vi "SetADGainGUI.vi"() -> ()   [LabVIEW 8.6]
uses:
  Program Files/National Instruments/LabVIEW 2010/resource/objmgr/daqmx.rc
panel:
  in  "select AI range":u16(ring) items=["-0.2 : 0.2 V", "-0.5 : 0.5 V", "-1.0 : 1.0 V", "-2.0 : 2.0 V", "-5.0 : 5.0 V", "-10.0 : 10.0 V", "-20.0 : 20.0 V", "-42.0 : 42.0 V"]
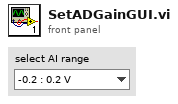
[diagram p1: front panel]
types:
  T1 = enum16{"None/#Datasets", "Clear", "TagValueOf#", "AddValues", "ReadValue", "ChangeValue", "Get all"}
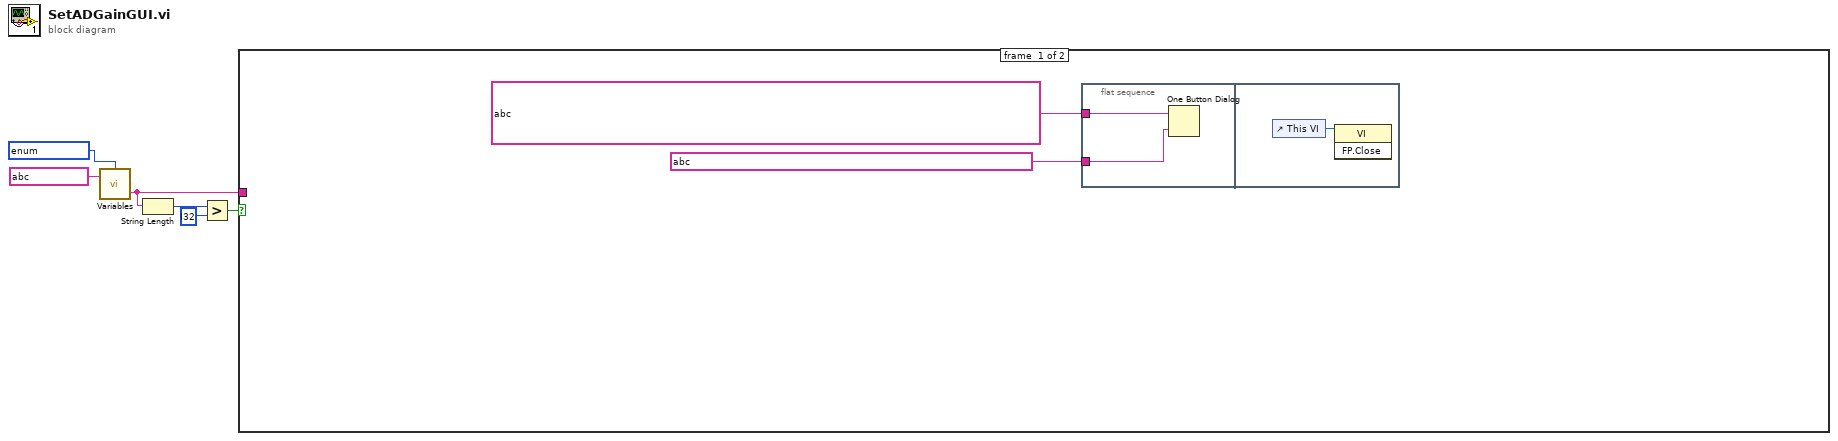
[diagram p0: block diagram]
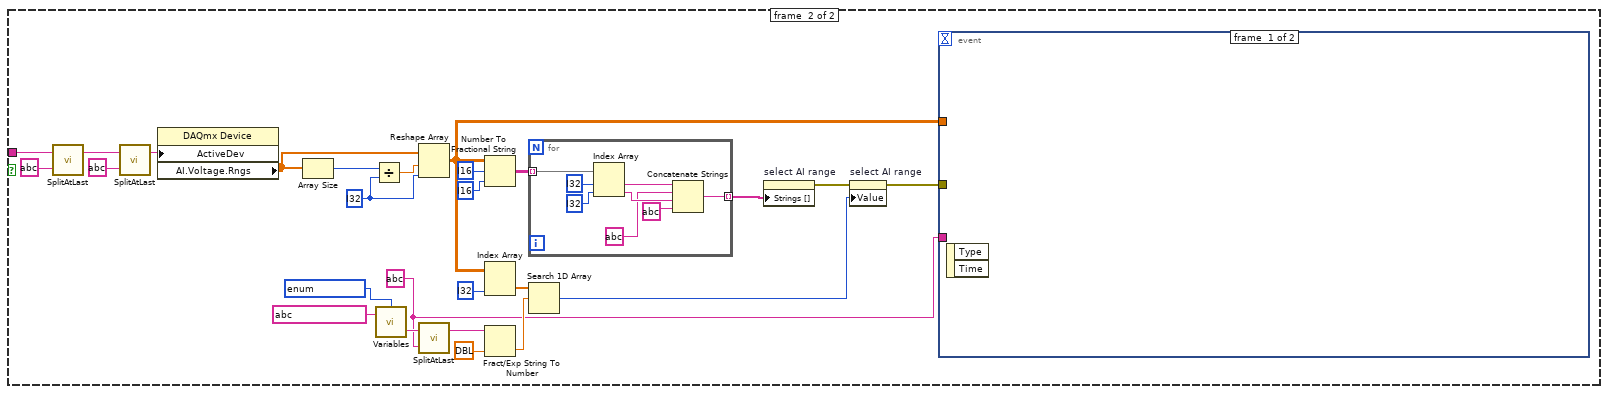
[diagram p2: hidden frame]
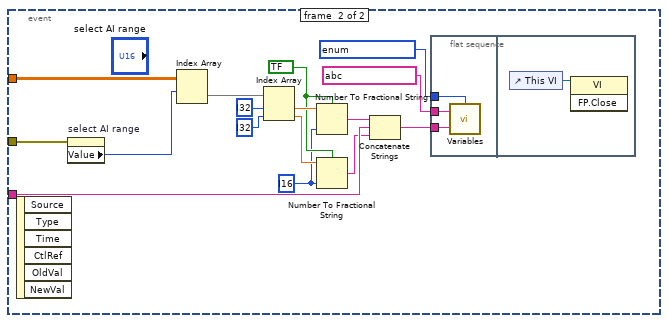
[diagram p3: hidden frame]
diagram:
  n1 = call "Variables.vi"("Tag in"=string ?, "Command"=T1 ?) -> ("value out"=w4:string)  [unwired: 1 in, 2 out]
  n2 = String Length(string=w4) -> (length=w3:i32)
  n3 = Greater?(x=w3, y=i32 ?) -> (0:w1:bool)
  n4 = case shown="True" w1 {
    tunnel: w4 -> [_ w12]
    frame #0 {
      n5 = flat-sequence {
        tunnel: string ? ("message") -> [w10]
        tunnel: string ? ("button name (\"OK\")") -> [w9]
        frame #0 {
          n6 = One Button Dialog(message=w10, button name ("OK")=w9) -> ()  [unwired: 1 out]
        }
        frame #1 {
          n7 = control-ref of="This VI"() -> (w11:refnum<vi>)
          n8 = invoke class="VI" method="FP.Close"(reference=w11) -> ()  [unwired: 2 in, 3 out]
        }
      }
    }
    frame #1 {
      w28 = i32 ? ("y")
      w13 = string ? ("search char")
      n9 = call "SplitAtLast.vi"("search char"=string ?, "In-String"=w12) -> ("Front (default)"=w36:string)  [unwired: 1 out]
      n10 = call "SplitAtLast.vi"("search char"=string ?, "In-String"=w36) -> ("Front (default)"=w34:string)  [unwired: 1 out]
      n11 = property class="DAQmx Device"("ActiveDev"=w34) -> ("AI.Voltage.Rngs"=w30:dbl[])  [unwired: 2 in, 2 out]
      n12 = Array Size(array=w30) -> (size(s)=w29:i32)
      n13 = Divide(x=w29, y=w28) -> (x/y=w27:dbl)
      n14 = call "Variables.vi"("Tag in"=string ?, "Command"=T1 ?) -> ("value out"=w31:string)  [unwired: 1 in, 2 out]
      n15 = Reshape Array(w30, w27, w28) -> (w14:dbl[][])
      n16 = call "SplitAtLast.vi"("search char"=w13, "In-String"=w31) -> ("Front (default)"=w22:string)  [unwired: 1 out]
      n17 = Number To Fractional String(number=w14, width (-)=i16 ?, precision (6)=i16 ?) -> (F-format string=w24:string[][])  [unwired: 1 out]
      n18 = Index Array(array=w14, index (col)=i32 ? ("disabled index (col)")) -> (element=w19:dbl[])  [unwired: 1 in]
      n19 = Fract/Exp String To Number(string=w22, default (0 dbl)=dbl ? ("default (0 I32)")) -> (number=w18:dbl)  [unwired: 3 out]
      n20 = for {
        tunnel: w24 -> [w45] mode=indexing
        tunnel: [w39] -> w23 mode=indexing
        n21 = Index Array(array=w45, index #1=i32 ? ("index"), index #2=i32 ? ("index")) -> (element #1=w42:string, element #2=w41:string)
        n22 = Concatenate Strings(w42, string ? ("string"), w41, string ? ("string")) -> (w39:string)
      }
      n23 = Search 1D Array(1D array=w19, element=w18) -> (index of element=w16:i32)  [unwired: 1 out]
      n24 = property on="select AI range" class="Ring (strict)"("Strings []"=w23) -> (error out=w17:errorcluster)  [unwired: 2 in, 1 out]
      n25 = property on="select AI range" class="Ring (strict)"(error in=w17, "Value"=w16) -> (error out=w15:errorcluster)  [unwired: 1 in, 1 out]
      n26 = event shown="[1] \"select AI range\": Value Change" {
        selector: _ -> [_ _]
        dyn-events: _ -> [_ _]
        timeout: _ -> [_ _]
        tunnel: w15 -> [_ w61]
        tunnel: w14 -> [_ w59]
        tunnel: w13 -> [_ w50]
        event #0 {
          n27 = event-data() -> ()  [unwired: 3 out]
        }
        event #1 {
          w52 = i16 ? ("precision (6)")
          w53 = bool ? ("use system decimal point (T)")
          n28 = event-data() -> ()  [unwired: 7 out]
          n29 = property on="select AI range" class="Ring (strict)"(error in=w61) -> ("Value"=w60:u16)  [unwired: 1 in, 2 out]
          n30 = Index Array(array=w59, index (row)=w60) -> (element=w58:dbl[])  [unwired: 1 in]
          n31 = Index Array(array=w58, index #1=i32 ? ("index"), index #2=i32 ? ("index")) -> (element #1=w55:dbl, element #2=w54:dbl)
          n32 = Number To Fractional String(use system decimal point (T)=w53, number=w55, precision (6)=w52) -> (F-format string=w51:string)  [unwired: 1 out]
          n33 = Number To Fractional String(use system decimal point (T)=w53, number=w54, precision (6)=w52) -> (F-format string=w49:string)  [unwired: 1 out]
          n34 = Concatenate Strings(w51, w50, w49) -> (w46:string)
          n35 = flat-sequence {
            tunnel: string ? ("Tag in") -> [w64]
            tunnel: T1 ? ("Command") -> [w63]
            tunnel: w46 -> [w62]
            frame #0 {
              n36 = call "Variables.vi"("value"=w62, "Tag in"=w64, "Command"=w63) -> ()  [unwired: 3 out]
            }
            frame #1 {
              n37 = control-ref of="This VI"() -> (w65:refnum<vi>)
              n38 = invoke class="VI" method="FP.Close"(reference=w65) -> ()  [unwired: 2 in, 3 out]
            }
          }
        }
      }
    }
  }
